vi "Task Construct2.vi"() -> ()   [LabVIEW 2015]
uses:
  Controls/Sample Transfer Container Enumerator.ctl
  Controls/Sample Transfer State Enumerator.ctl
  Controls/Sample Push State Enumerator.ctl
  Controls/Sample Transfer Control Enumerator.ctl
  Controls/Sample Push Control Enumerator.ctl
panel:
  in  "Sample Push Control":T1
  in  "Sample Transfer Control":T2
  out "Sample Push State":T3
  out "Sample Transfer State":T4
  in  "Target Container":T5
  in  "Source Container":T5
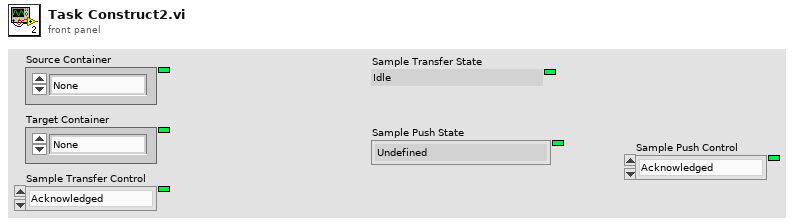
[diagram p1: front panel]
types:
  T1 = typedef "Sample Push Control Enumerator.ctl" = enum16{"Acknowledged", "Push", "Stash", "Abort", "Reset to Idle"}
  T2 = typedef "Sample Transfer Control Enumerator.ctl" = enum16{"Acknowledged", "Transfer", "Stash", "Abort", "Reset to Idle"}
  T3 = typedef "Sample Push State Enumerator.ctl" = enum16{"Undefined", "Initialize", "Dilute", "Close Transfer Line", "Start Heaters", "Warm Up Syringe", "Ready to Push", "Push", "Initiate Stash", "Stash", "Complete", "Abort", "Idle", "Error"}
  T4 = typedef "Sample Transfer State Enumerator.ctl" = enum16{"Idle", "Initialize", "Check Containers", "Check Temperatures", "Start Turbo", "Warm Up Containers", "Prepare for purging", "Purge Capillary", "Purge", "Open Containers", "Introduce Sample", "Measure Base Pressure", "Home Syringe", "Start Freezer", "Freeze Target", "Crystalize", "Initiate Stash", "Stash", "Polish", "Stop Freezers", "Push Sample", "Complete", "Abort", "Error", "Undefined"}
  T5 = typedef "Sample Transfer Container Enumerator.ctl" = enum16{"None", "Sample 1", "Sample 2", "Sample 3", "Sample 4", "Sample 5", "Storage 01", "Storage 02", "Storage 03", "Storage 04", "Storage 05", "Storage 06", "Storage 07", "Storage 08", "Storage 09", "Storage 10", "Storage 11", "Storage 12", "Syringe", "Undefined"}
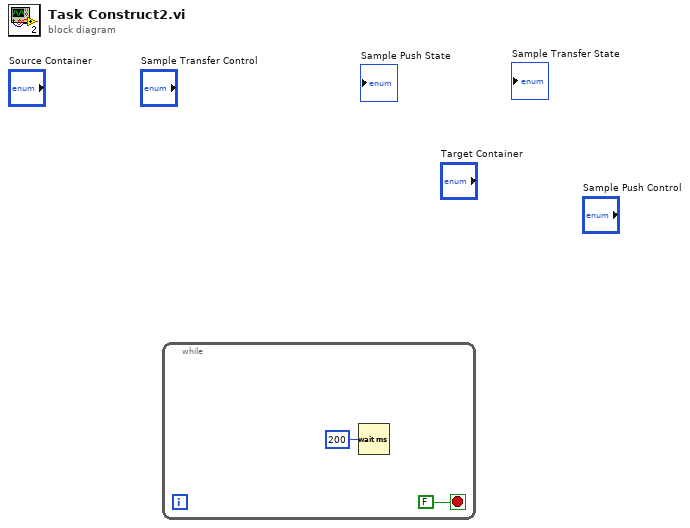
[diagram p0: block diagram]
diagram:
  n1 = while {
    stop <- FALSE stop-if-true
    n2 = Wait (ms)(milliseconds to wait=u32 200) -> ()  [unwired: 1 out]
  }
